vi "Select myDAQ Device.vi"(8 "Error In":errorcluster, 11 "ProductType":string="NI myDAQ") -> (0 "Error Out":errorcluster, 3 "DAQmx Device Name":tag)   [LabVIEW 2017]
uses:
  <resource>/objmgr/daqmx.rc
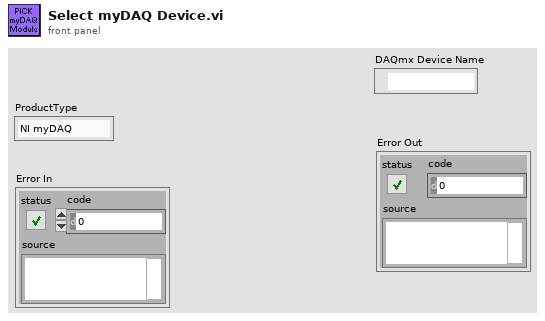
[diagram p1: front panel]
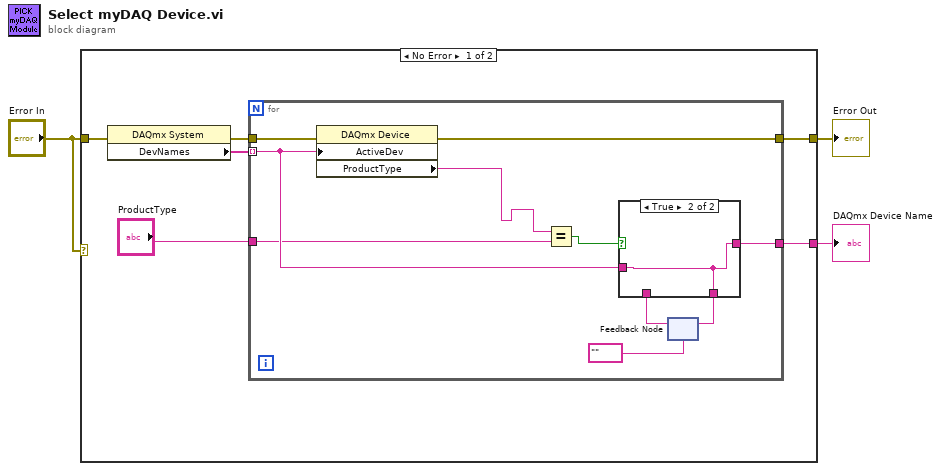
[diagram p0: block diagram]
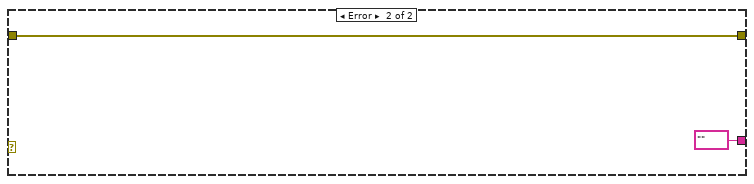
[diagram p3: hidden frame]
diagram:
  n1 = case shown="No Error" "Error In" {
    tunnel: [w7 tag ""] -> w3
    tunnel: [w6 w23] -> w2
    tunnel: "Error In" -> [w4 w23]
    frame No Error {
      n2 = property class="DAQmx System"(error in=w4) -> (error out=w9:errorcluster, "DevNames"=w8:tag[])  [unwired: 1 in, 1 out]
      n3 = for {
        tunnel: w9 -> [w19]
        tunnel: w8 -> [w16] mode=indexing
        tunnel: [w12] -> w7
        tunnel: [w11] -> w6
        tunnel: "ProductType" -> [w10]
        n4 = property class="DAQmx Device"(error in=w19, "ActiveDev"=w16) -> (error out=w11:errorcluster, "ProductType"=w18:string)  [unwired: 1 in, 1 out]
        n5 = Equal?(x=w18, y=w10) -> (x = y?=w17:bool)
        n6 = feedback #1(tag "") -> (w13:tag)
        n7 = case shown="True" w17 {
          tunnel: w16 -> [_ w21]
          tunnel: [w20 w21] -> w15
          tunnel: w13 -> [w20 _]
          tunnel: [w20 w21] -> w12
          frame False {
          }
          frame True {
          }
        }
        n8 = feedback-in #1(w15) -> ()
      }
    }
    frame Error {
    }
  }
  "DAQmx Device Name" <- w3
  "Error Out" <- w2
